vi "Sample Rate To Loop Time (ticks).vi"(0 "sample rate (S/s)":dbl format="%#_6p", 1 "FPGA clock rate (Hz)":dbl=40000000.0 format="%#_6p", 11 "error in (no error)":errorcluster) -> (4 "count (ticks/S)":u32, 10 "actual sample rate (S/s)":dbl format="%#_6p", 15 "error out":errorcluster)   [LabVIEW 2017, in "NI_FpgaMspHost.lvlib"]
doc: "Converts the desired sample rate to the appropriate count for the Loop Timer Express VI and computes the achievable sample rate for use with other Scaling VIs."
uses:
  <vilib>/rvi/Analysis/host/Public/NI_FpgaMspHost.lvlib
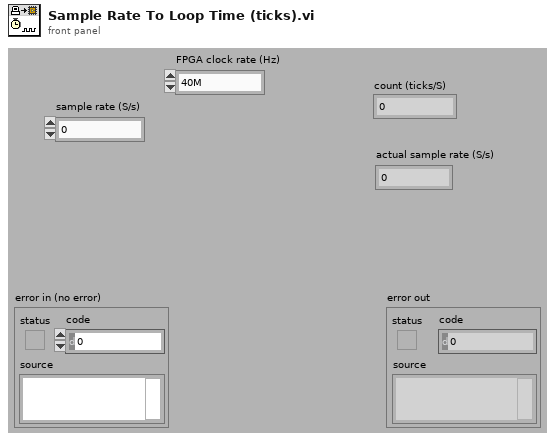
[diagram p1: front panel]
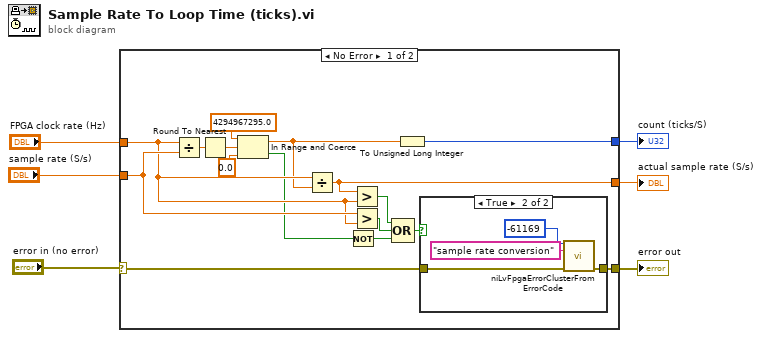
[diagram p0: block diagram]
diagram:
  n1 = case shown="No Error" "error in (no error)" {
    selector: "error in (no error)" -> [w20 w28]
    tunnel: "FPGA clock rate (Hz)" -> [w14 _]
    tunnel: "sample rate (S/s)" -> [w15 _]
    tunnel: [w21 _] -> w3
    tunnel: [w16 _] -> w2
    tunnel: [w19 w28] -> w1
    frame No Error {
      n2 = Divide(x=w14, y=w15) -> (x/y=w9:dbl)
      n3 = Round To Nearest(number=w9) -> (nearest integer value=w10:dbl)
      n4 = In Range and Coerce(upper limit=4294967295.0 ("unsigned 32bit integer"), x=w10, lower limit=0.0) -> (coerced(x)=w7:dbl, In Range?=w8:bool)
      n5 = Divide(x=w14, y=w7) -> (x/y=w16:dbl)
      n6 = Not(x=w8) -> (.not. x?=w18:bool)
      n7 = Greater?(x=w16, y=w14) -> (0:w17:bool)
      n8 = Greater?(x=w15, y=w14) -> (0:w13:bool)
      n9 = Compound Arithmetic op=OR(w17, w13, w18) -> (w22:bool)
      n10 = To Unsigned Long Integer(number=w7) -> (unsigned 32bit integer=w21:u32)
      n11 = case shown="True" w22 {
        tunnel: [w23 w27] -> w19
        tunnel: w20 -> [w23 w24]
        frame False {
        }
        frame True {
          n12 = call <vilib>:"niLvFpgaErrorClusterFromErrorCode.vi"("error code"=-61169, "function name"="sample rate conversion" ("L10N_Function Name"), "error in"=w24) -> ("error out"=w27:errorcluster)  [unwired: 4 in, 8 out]
        }
      }
    }
    frame Error {
    }
  }
  "error out" <- w1
  "count (ticks/S)" <- w3
  "actual sample rate (S/s)" <- w2
